vi "NewBombedMazeGame.vi"(8 "error in (no error)":errorcluster) -> (0 "error out":errorcluster, 3 "BombedMazeGame":refnum<class "BombedMazeGame.lvclass">)   [LabVIEW 2020, in "FactoryMethod.lvlib" / "NoParametrizedFactoryMethod.lvlib" / "BombedMazeGame.lvclass"]
uses:
  BombedMazeGame.lvclass
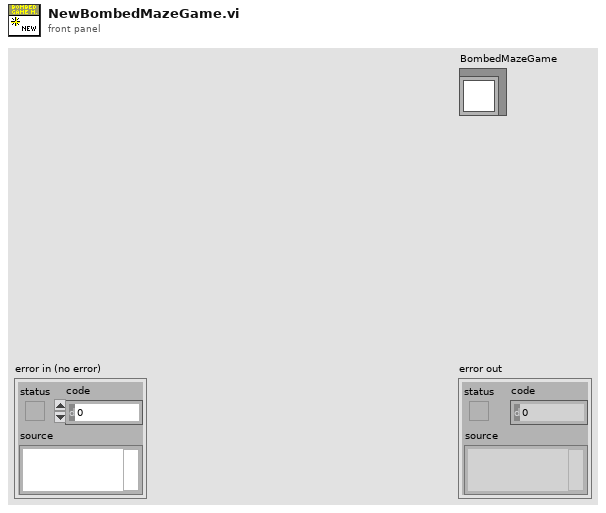
[diagram p1: front panel]
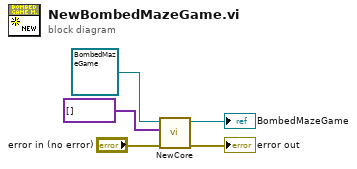
[diagram p0: block diagram]
diagram:
  n1 = call-dynamic "NewCore.vi"("error in (no error)"="error in (no error)", "ParamsArray"=variant[] [], "BombedMazeGame"=refnum<class "BombedMazeGame.lvclass"> refnum ("ByRef")) -> ("error out"=→"error out":errorcluster, "BombedMazeGame"=→"BombedMazeGame":refnum<class "BombedMazeGame.lvclass">)  [unwired: 7 in]
